vi "InputProc.vi"(8 "Sensors":cluster{T2[], T6[], T7[], T9[]}, 9 "Gamepad Data":T11, 10 "SensorInputData":T12) -> (2 "Gamepad Data Out":T11, 3 "SensorInputDataOut":T12)   [LabVIEW 2015]
uses:
  Typedefs/SensorInputData.ctl
  Typedefs/GamepadData.ctl
  <vilib>/Rock Robotics/WPI/Encoder/WPI_EncoderDevRef.ctl
  <vilib>/Rock Robotics/SystemInterfaces/Encoder/FPGA_EncoderIdx.ctl
  <vilib>/Rock Robotics/SystemInterfaces/Counter/FPGA_CounterCtrSystemIndex.ctl
  <vilib>/Rock Robotics/WPI/Encoder/WPI_EncoderType.ctl
  <vilib>/Rock Robotics/WPI/Counter/WPI_CounterDevRef.ctl
  <vilib>/Rock Robotics/WPI/Switch/WPI_SwitchDevRef.ctl
  <vilib>/Rock Robotics/SystemInterfaces/DIO/FPGA_DIOChannel.ctl
  <vilib>/Rock Robotics/WPI/Potentiometer/WPI_PotentiometerDevRef.ctl
  <vilib>/Rock Robotics/SystemInterfaces/AI/FPGA_AIChannel.ctl
  Typedefs/JoysticksGlobal.vi
panel:
  in  "Hood Position Inputs":T1
  in  "Collector Lift Inputs":T1
  in  "ENC_CPR":dbl format="%#_13g"
  in  "ENC_CPI":dbl format="%#_13g"
  # "For Shooter"
  # "For Drivetrain"
  # "is now f310"
  # "ENC_CPI is encoder counts per inch"
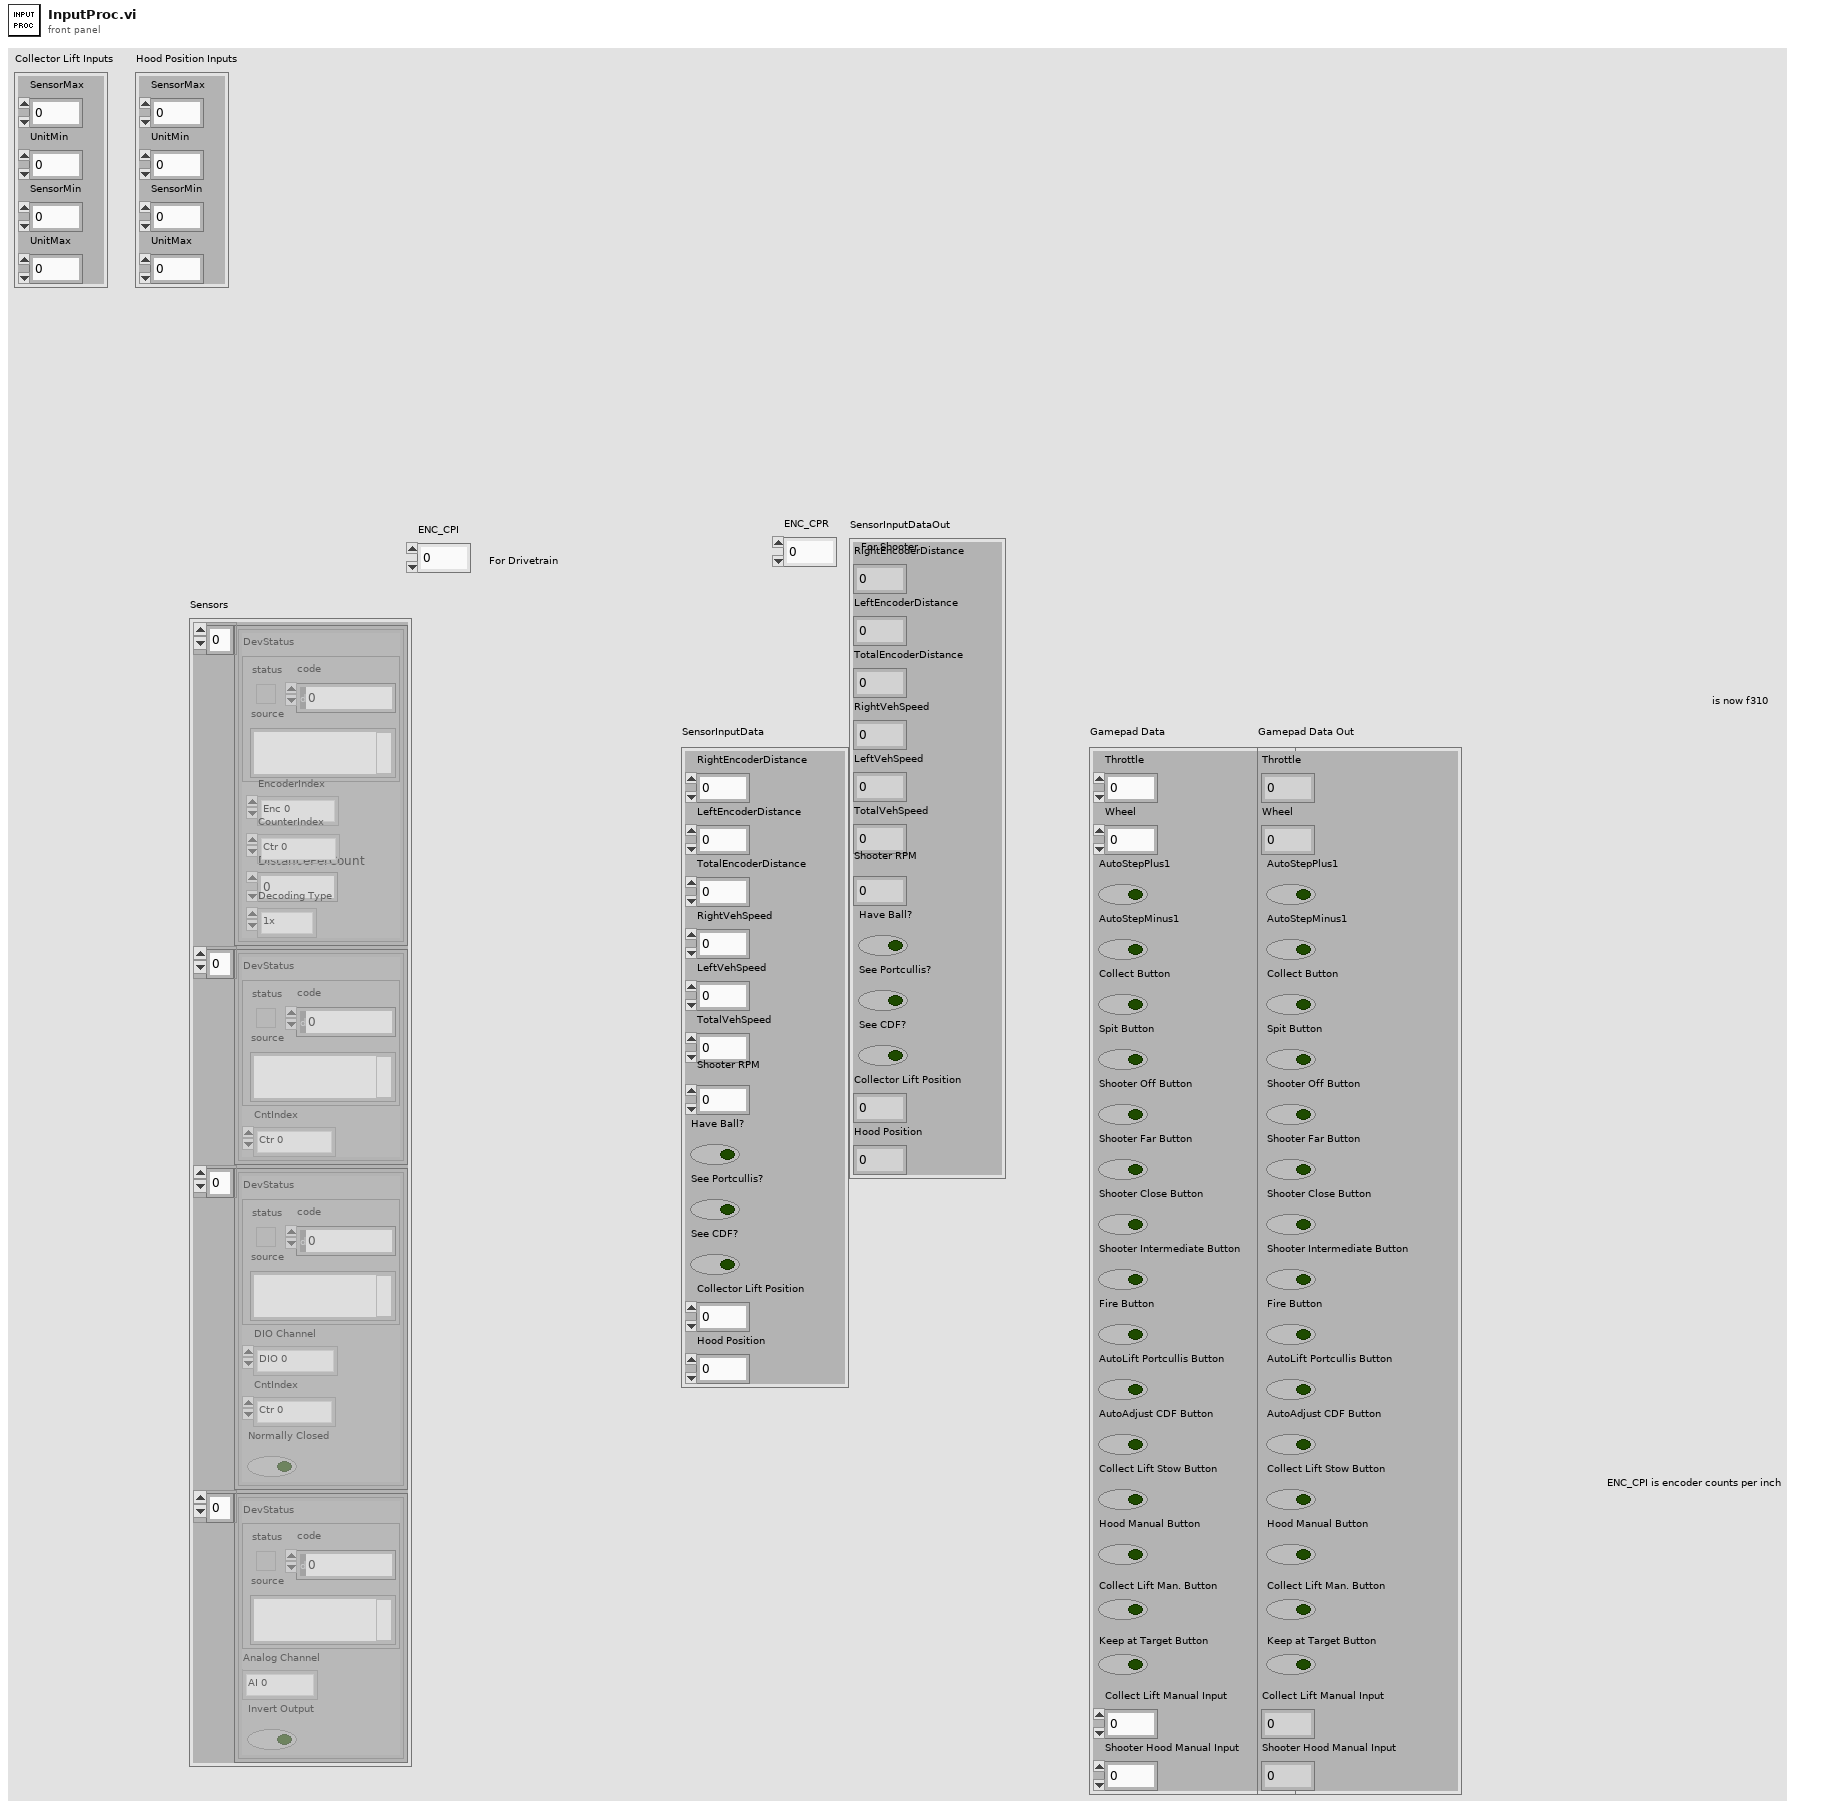
[diagram p1: front panel]
types:
  T1 = cluster{"SensorMax":dbl, "UnitMin":dbl, "SensorMin":dbl, "UnitMax":dbl}
  T2 = typedef "WPI_EncoderDevRef.ctl" = cluster{"DevStatus":errorcluster, "EncoderIndex":T3, "CounterIndex":T4, "DistancePerCount":dbl, "Decoding Type":T5}
  T3 = typedef "FPGA_EncoderIdx.ctl" = enum8{"Enc 0", "Enc 1", "Enc 2", "Enc 3", "Enc 4", "Enc 5", "Enc 6", "Enc 7", "Invalid"}
  T4 = typedef "FPGA_CounterCtrSystemIndex.ctl" = enum8{"Ctr 0", "Ctr 1", "Ctr 2", "Ctr 3", "Ctr 4", "Ctr 5", "Ctr 6", "Ctr 7", "Invalid"}
  T5 = typedef "WPI_EncoderType.ctl" = enum16{"1x", "2x", "4x"}
  T6 = typedef "WPI_CounterDevRef.ctl" = cluster{"DevStatus":errorcluster, "CntIndex":T4}
  T7 = typedef "WPI_SwitchDevRef.ctl" = cluster{"DevStatus":errorcluster, "DIO Channel":T8, "CntIndex":T4, "Normally Closed":bool}
  T8 = typedef "FPGA_DIOChannel.ctl" = enum8{"DIO 0", "DIO 1", "DIO 2", "DIO 3", "DIO 4", "DIO 5", "DIO 6", "DIO 7", "DIO 8", "DIO 9", "DIO MXP 0", "DIO MXP 1", "DIO MXP 2", "DIO MXP 3", "DIO MXP 4", "DIO MXP 5", "DIO MXP 6", "DIO MXP 7", "DIO MXP 8", "DIO MXP 9", "DIO MXP 10", "DIO MXP 11", "DIO MXP 12", "DIO MXP 13", "DIO MXP 14", "DIO MXP 15", "Invalid"}
  T9 = typedef "WPI_PotentiometerDevRef.ctl" = cluster{"DevStatus":errorcluster, "Analog Channel":T10, "Invert Output":bool}
  T10 = typedef "FPGA_AIChannel.ctl" = enum8{"AI 0", "AI 1", "AI 2", "AI 3", "AI MXP 0", "AI MXP 1", "AI MXP 2", "AI MXP 3", "Invalid"}
  T11 = typedef "GamepadData.ctl" = cluster{"Throttle":dbl, "Wheel":dbl, "AutoStepPlus1":bool, "AutoStepMinus1":bool, "Collect Button":bool, "Spit Button":bool, "Shooter Off Button":bool, "Shooter Far Button":bool, "Shooter Close Button":bool, "Shooter Intermediate Button":bool, "Fire Button":bool, "AutoLift Portcullis Button":bool, "AutoAdjust CDF Button":bool, "Collect Lift Stow Button":bool, "Hood Manual Button":bool, "Collect Lift Man. Button":bool, "Keep at Target Button":bool, "Collect Lift Manual Input":dbl, "Shooter Hood Manual Input":dbl}
  T12 = typedef "SensorInputData.ctl" = cluster{"RightEncoderDistance":dbl, "LeftEncoderDistance":dbl, "TotalEncoderDistance":dbl, "RightVehSpeed":dbl, "LeftVehSpeed":dbl, "TotalVehSpeed":dbl, "Shooter RPM":dbl, "Have Ball?":bool, "See Portcullis?":bool, "See CDF?":bool, "Collector Lift Position":dbl, "Hood Position":dbl}
  T13 = cluster{cluster{"Axes":dbl[], "Buttons":bool[], "POVs":i16[]}, cluster{"Axes":dbl[], "Buttons":bool[], "POVs":i16[]}}
  T14 = cluster{"Axes":dbl[], "Buttons":bool[], "POVs":i16[]}
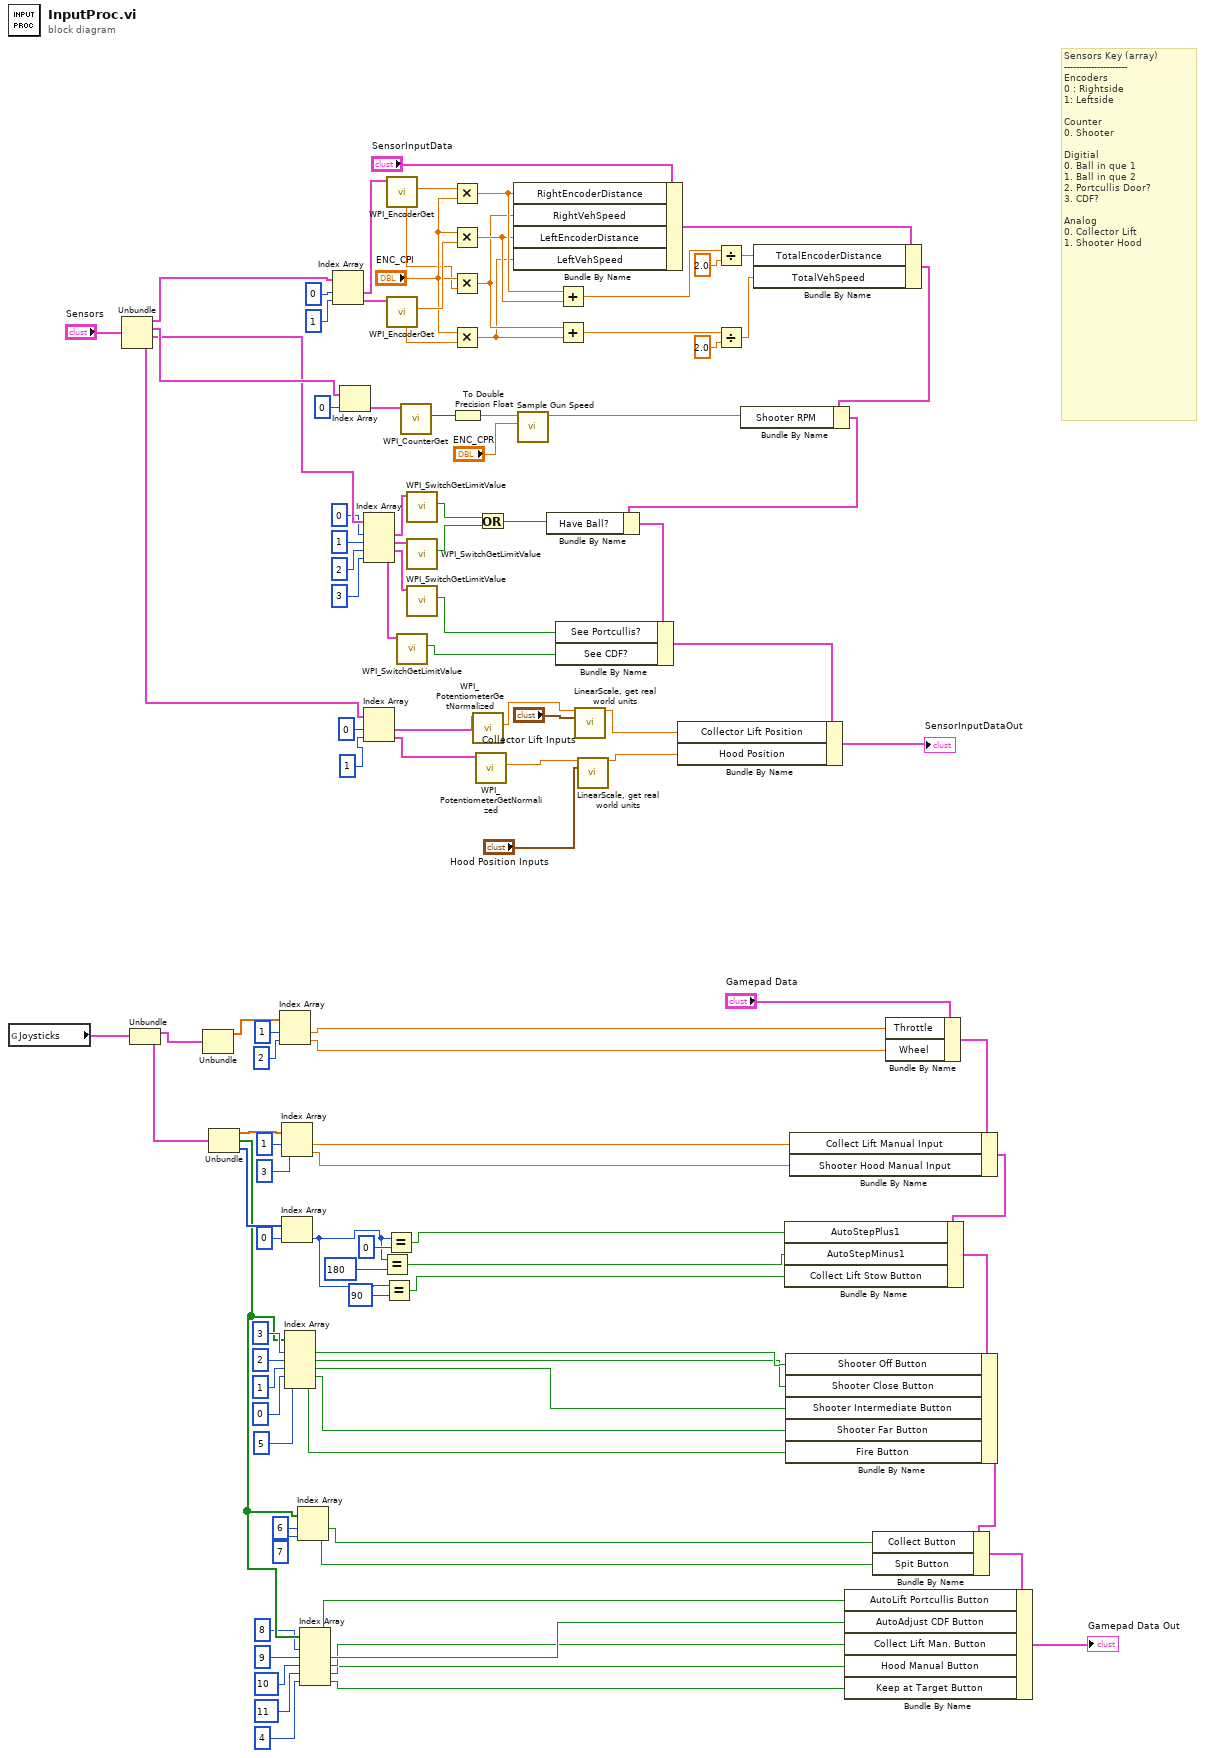
[diagram p0: block diagram]
diagram:
  # "Sensors Key (array)\n---------------------\nEncoders\n0 : Rightside\n1: Leftside\n\nCounter\n0. Shooter\n\nDigitial\n0. Ball in que 1\n1. Ball in que 2\n2. Portcullis Door?\n3. CDF?\n\nAnalog\n0. Collector Lift\n1. Shooter Hood"
  n1 = global read "JoysticksGlobal.vi" "Joysticks"() -> (w49:T13)
  n2 = Unbundle("Sensors") -> (w79:T2[], w76:T6[], w74:T7[], w58:T9[])
  n3 = Unbundle(w49) -> (w46:T14, w40:T14)
  n4 = Unbundle(w46) -> ("Axes"=w45:dbl[])  [unwired: 2 out]
  n5 = Unbundle(w40) -> ("Axes"=w39:dbl[], "Buttons"=w11:bool[], "POVs"=w34:i16[])
  n6 = Index Array(array=w45, index #1=1 ("index"), index #2=2 ("index")) -> (element #1=w43:dbl, element #2=w41:dbl)
  n7 = Index Array(array=w39, index #1=1 ("index"), index #2=3 ("index")) -> (element #1=w37:dbl, element #2=w35:dbl)
  n8 = Index Array(array=w34, index=0) -> (element=w28:i16)
  n9 = Index Array(array=w11, index #1=3 ("index"), index #2=2 ("index"), index #3=1 ("index"), index #4=0 ("index"), index #5=5 ("index")) -> (element #1=w24:bool, element #2=w23:bool, element #3=w21:bool, element #4=w18:bool, element #5=w16:bool)
  n10 = Index Array(array=w11, index #1=6 ("index"), index #2=7 ("index")) -> (element #1=w13:bool, element #2=w12:bool)
  n11 = Index Array(array=w11, index #1=8 ("index"), index #2=9 ("index"), index #3=10 ("index"), index #4=11 ("index"), index #5=4 ("index")) -> (element #1=w9:bool, element #2=w7:bool, element #3=w5:bool, element #4=w3:bool, element #5=w1:bool)
  n12 = Index Array(array=w79, index #1=0 ("index"), index #2=1 ("index")) -> (element #1=w78:T2, element #2=w77:T2)
  n13 = Index Array(array=w76, index=0) -> (element=w75:T6)
  n14 = Index Array(array=w74, index #1=0 ("index"), index #2=1 ("index"), index #3=2 ("index"), index #4=3 ("index")) -> (element #1=w72:T7, element #2=w68:T7, element #3=w64:T7, element #4=w61:T7)
  n15 = Index Array(array=w58, index #1=0 ("index"), index #2=1 ("index")) -> (element #1=w57:T9, element #2=w56:T9)
  n16 = Equal?(x=w28, y=i16 180) -> (x = y?=w29:bool)
  n17 = Equal?(x=w28, y=i16 90) -> (x = y?=w26:bool)
  n18 = Equal?(x=w28, y=i16 0) -> (x = y?=w31:bool)
  n19 = call <vilib>:"WPI_EncoderGet.vi"("EncoderDevRef"=w78) -> ("Distance"=w101:dbl, "Rate"=w92:dbl)  [unwired: 5 in, 4 out]
  n20 = call <vilib>:"WPI_EncoderGet.vi"("EncoderDevRef"=w77) -> ("Distance"=w100:dbl, "Rate"=w93:dbl)  [unwired: 5 in, 4 out]
  n21 = call <vilib>:"WPI_SwitchGetLimitValue.vi"("SwitchDevRef"=w61) -> ("Switch Pressed"=w62:bool)  [unwired: 8 in, 2 out]
  n22 = call <vilib>:"WPI_CounterGet.vi"("CounterDevRef in"=w75) -> ("Value"=w85:i32)  [unwired: 5 in, 5 out]
  n23 = call <vilib>:"WPI_SwitchGetLimitValue.vi"("SwitchDevRef"=w72) -> ("Switch Pressed"=w67:bool)  [unwired: 8 in, 2 out]
  n24 = call <vilib>:"WPI_SwitchGetLimitValue.vi"("SwitchDevRef"=w68) -> ("Switch Pressed"=w66:bool)  [unwired: 8 in, 2 out]
  n25 = call <vilib>:"WPI_SwitchGetLimitValue.vi"("SwitchDevRef"=w64) -> ("Switch Pressed"=w63:bool)  [unwired: 8 in, 2 out]
  n26 = Multiply(x=w101, y="ENC_CPI") -> (x*y=w91:dbl)
  n27 = Multiply(x="ENC_CPI", y=w100) -> (x*y=w90:dbl)
  n28 = Multiply(x="ENC_CPI", y=w92) -> (x*y=w89:dbl)
  n29 = Multiply(x="ENC_CPI", y=w93) -> (x*y=w87:dbl)
  n30 = To Double Precision Float(number=w85) -> (double precision float=w84:dbl)
  n31 = call <vilib>:"WPI_PotentiometerGetNormalized.vi"("PotDevRef"=w57) -> ("Normalized Value"=w54:dbl)  [unwired: 8 in, 2 out]
  n32 = call <vilib>:"WPI_PotentiometerGetNormalized.vi"("PotDevRef"=w56) -> ("Normalized Value"=w51:dbl)  [unwired: 8 in, 2 out]
  n33 = Or(x=w67, y=w66) -> (x .or. y?=w65:bool)
  n34 = Bundle By Name(cluster="SensorInputData", "RightEncoderDistance"=w91, "RightVehSpeed"=w89, "LeftEncoderDistance"=w90, "LeftVehSpeed"=w87) -> (w102:T12)
  n35 = call "Sample Gun Speed.vi"("Encoder Counts per Rotation"="ENC_CPR", "Shooter Rotations"=w84) -> ("Shooter RPM"=w81:dbl)  [unwired: 9 in]
  n36 = Add(x=w91, y=w90) -> (x+y=w98:dbl)
  n37 = Add(x=w89, y=w87) -> (x+y=w95:dbl)
  n38 = call "LinearScale, get real world units.vi"("RawInput"=w54, "UnitsPlease Inputs"="Collector Lift Inputs") -> ("UnitOutput"=w53:dbl)  [unwired: 13 in]
  n39 = call "LinearScale, get real world units.vi"("RawInput"=w51, "UnitsPlease Inputs"="Hood Position Inputs") -> ("UnitOutput"=w50:dbl)  [unwired: 13 in]
  n40 = Divide(x=w98, y=2.0) -> (x/y=w97:dbl)
  n41 = Divide(x=w95, y=2.0) -> (x/y=w88:dbl)
  n42 = Bundle By Name(cluster=w102, "TotalEncoderDistance"=w97, "TotalVehSpeed"=w88) -> (w82:T12)
  n43 = Bundle By Name(cluster=w82, "Shooter RPM"=w81) -> (w107:T12)
  n44 = Bundle By Name(cluster=w107, "Have Ball?"=w65) -> (w106:T12)
  n45 = Bundle By Name(cluster=w106, "See Portcullis?"=w63, "See CDF?"=w62) -> (w105:T12)
  n46 = Bundle By Name(cluster=w105, "Collector Lift Position"=w53, "Hood Position"=w50) -> (→"SensorInputDataOut":T12)
  n47 = Bundle By Name(cluster="Gamepad Data", "Throttle"=w43, "Wheel"=w41) -> (w47:T11)
  n48 = Bundle By Name(cluster=w47, "Collect Lift Manual Input"=w37, "Shooter Hood Manual Input"=w35) -> (w109:T11)
  n49 = Bundle By Name(cluster=w109, "AutoStepPlus1"=w31, "AutoStepMinus1"=w29, "Collect Lift Stow Button"=w26) -> (w114:T11)
  n50 = Bundle By Name(cluster=w114, "Shooter Off Button"=w24, "Shooter Close Button"=w23, "Shooter Intermediate Button"=w21, "Shooter Far Button"=w18, "Fire Button"=w16) -> (w113:T11)
  n51 = Bundle By Name(cluster=w113, "Collect Button"=w13, "Spit Button"=w12) -> (w111:T11)
  n52 = Bundle By Name(cluster=w111, "AutoLift Portcullis Button"=w9, "AutoAdjust CDF Button"=w7, "Collect Lift Man. Button"=w5, "Hood Manual Button"=w3, "Keep at Target Button"=w1) -> (→"Gamepad Data Out":T11)
